vi "Get Monotonic Time.vi"(11 "Generic Network Address in":refnum<class "Generic Network Address.lvclass">) -> (2 "timestamp":u32, 3 "Generic Network Address out":refnum<class "Generic Network Address.lvclass">)   [LabVIEW 2020, in "NI_WFCN.lvlib" / "Generic Network Address.lvclass"]
doc: "Returns a monotonically increasing timestamp value."
uses:
  <vilib>/net/WFCN/Addressing/Generic Network Address/Generic Network Address.lvclass
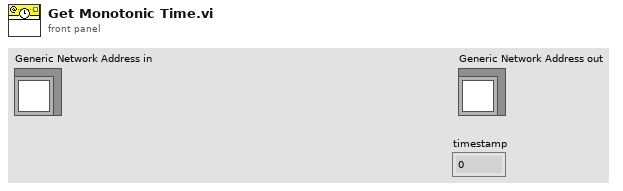
[diagram p1: front panel]
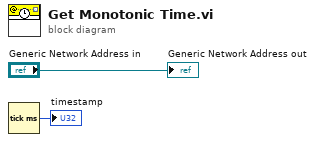
[diagram p0: block diagram]
diagram:
  n1 = Tick Count (ms)() -> (millisecond timer value=→"timestamp":u32)
  "Generic Network Address out" <- "Generic Network Address in"
